vi "DefaultConstructor.vi"(10 "ValueType":variant, 11 "KeyType":variant) -> (3 "Map":refnum<class "Map.lvclass">)   [LabVIEW 2016, in "Map.lvclass"]
uses:
  <userlib>/836-libraries/Data_Structures/Map/Map.lvclass
  <userlib>/836-libraries/Data_Structures/Map/Map.lvclass/Map.ctl
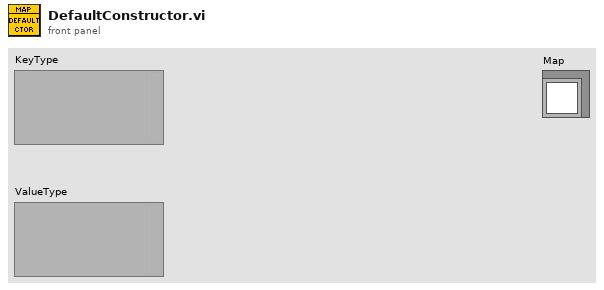
[diagram p1: front panel]
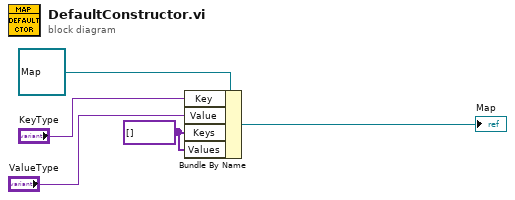
[diagram p0: block diagram]
diagram:
  w1 = variant[] [] ("Keys")
  n1 = Bundle By Name(cluster=refnum<class "Map.lvclass"> refnum ("Map"), "Key"="KeyType", "Value"="ValueType", "Keys"=w1, "Values"=w1) -> (→"Map":refnum<class "Map.lvclass">)
